vi "Check For New File.vi"(7 "user@host":string, 8 "error in (no error)":errorcluster, 10 "Previous file name":string, 11 "OpenSSH Client in":refnum<class "OpenSSH Client.lvclass">) -> (0 "error out":errorcluster, 2 "Next file name":string)   [LabVIEW 2021, in "VeriStand Console.lvlib"]
uses:
  VeriStand Console.lvlib
  <vilib>/net/SSH/Client/OpenSSH/OpenSSH Client.lvclass
  C:/Program Files/National Instruments/LabVIEW 2021/vi.lib/net/SSH/Client/Generic/Generic Client.lvclass
  <vilib>/net/SSH/NI_SSH.lvlib
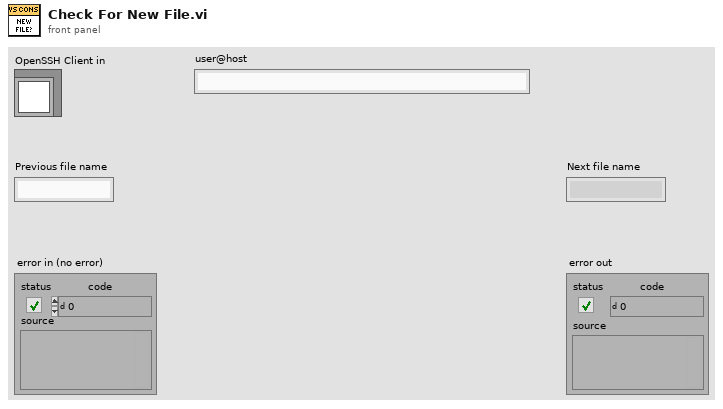
[diagram p1: front panel]
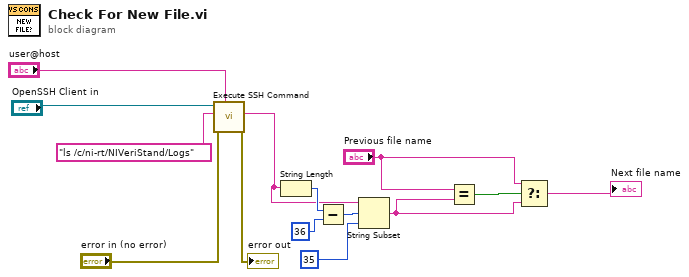
[diagram p0: block diagram]
diagram:
  n1 = call <vilib>:"Execute SSH Command.vi"("user@host"="user@host", "error in (no error)"="error in (no error)", "command line"="ls /c/ni-rt/NIVeriStand/Logs", "session in"="OpenSSH Client in") -> ("error out"=→"error out":errorcluster, "standard output"=w8:string)  [unwired: 3 in, 3 out]
  n2 = String Length(string=w8) -> (length=w11:i32)
  n3 = Subtract(x=w11, y=36) -> (x-y=w12:i32)
  n4 = String Subset(string=w8, offset (0)=w12, length (rest)=35 ("length (rest)")) -> (substring=w4:string)
  n5 = Equal?(x="Previous file name", y=w4) -> (x = y?=w7:bool)
  n6 = Select(t="Previous file name", s=w7, f=w4) -> (s? t:f=→"Next file name":string)
